vi "Clean Test Folder.vi"(4 "error in":errorcluster) -> (0 "error out":errorcluster)   [LabVIEW 2025]
doc: "This VI deletes the test folder and all its contents."
uses:
  <userlib>/_OpenG.lib/file/file.llb/openg_file.lvlib
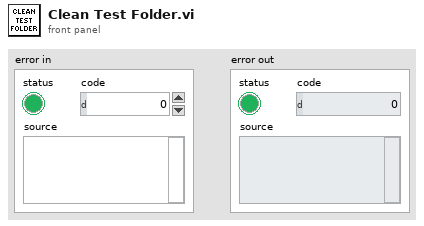
[diagram p1: front panel]
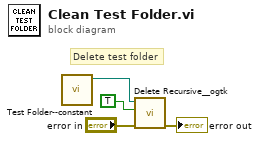
[diagram p0: block diagram]
diagram:
  # "Delete test folder"
  n1 = call "Test Folder--constant.vi"() -> ("Test Folder"=w1:path)  [unwired: 7 in]
  n2 = call <userlib>:"Delete Recursive__ogtk.vi"("error in (no error)"="error in", "Recursive? (FALSE)"=TRUE, "Path"=w1) -> ("error out"=→"error out":errorcluster)  [unwired: 7 in, 1 out]
